vi "MXA Configure AmplitudeWrite).vi"(0 "VISA resource name":refnum<visa-resource-name>="TCPIP0::169.254.70.120::inst0::INSTR", 11 "error in (no error)":errorcluster, 13 "Internal Preamp (0: Off)":i32(ring)=2 items=["Off", "Low Band", "Full Range"]) -> (4 "VISA resource name out":refnum<visa-resource-name>="TCPIP0::169.254.70.120::inst0::INSTR", 15 "error out":errorcluster)   [LabVIEW 2018]
doc: "Configures Preselector, Internal Preamp and Max Mixer Level."
uses:
  Agilent MXA Series/Agilent MXA Series.lvlib
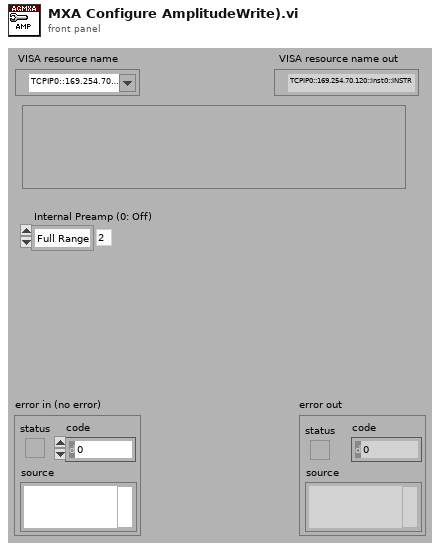
[diagram p1: front panel]
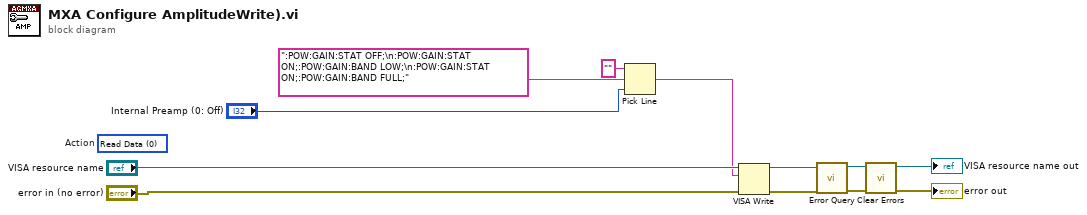
[diagram p0: block diagram]
diagram:
  (unwired) 0 items=["Read Data", "Write Data", "Clear Data", "Clear ALL Data"]  # Action
  n1 = Pick Line(string ("")="", multi-line string=":POW:GAIN:STAT OFF;\n:POW:GAIN:STAT ON;:POW:GAIN:BAND LOW;\n:POW:GAIN:STAT ON;:POW:GAIN:BAND FULL;", line index="Internal Preamp (0: Off)") -> (output string=w3:string)
  n2 = VISA Write(VISA resource name="VISA resource name", write buffer=w3, error in (no error)="error in (no error)") -> (VISA resource name out=w8:refnum<visa-resource-name>, error out=w9:errorcluster)  [unwired: 1 out]
  n3 = call "Error Query.vi"("error in (no error)"=w9, "VISA resource name"=w8) -> ("error out"=w6:errorcluster, "VISA resource name out"=→"VISA resource name out":refnum<visa-resource-name>)  [unwired: 6 in, 2 out]
  n4 = call <vilib>:"Clear Errors.vi"("error in (no error)"=w6) -> ("error out"=→"error out":errorcluster)  [unwired: 5 in, 1 out]
